vi "FRCts20_Backend_API_CompetitionRoot.vi"(8 "error in (no error)":errorcluster, 10 "Message":T1="GetCompetitionRoot") -> (0 "error out":errorcluster, 2 "Status":string, 3 "Competitions":T2)   [LabVIEW 2014]
doc: "This VI currently has just one command, which is to return all competitions. This cannot be rolled into another API VI, as no other VIs return competitions."
uses:
  FRCts20_Backend_API_CompetitionRoot.ctl
  FRCts20_Backend_API_Command_CompRoot.ctl
  FRCts20_Backend_FGVOperation.ctl
  FRCts20_Backend_Engine.lvlib
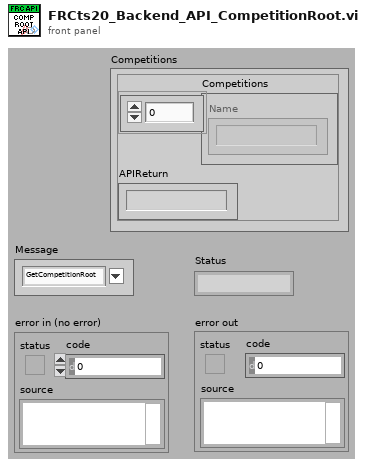
[diagram p1: front panel]
types:
  T1 = typedef "FRCts20_Backend_API_Command_CompRoot.ctl" = string
  T2 = typedef "FRCts20_Backend_API_CompetitionRoot.ctl" = cluster{"Competitions":string[], "APIReturn":string}
  T3 = typedef "FRCts20_Backend_Engine.lvlib/FRCts20_Backend_FGVOperation.ctl" = enum16{"Initialize", "EnqueueMessage", "EnqueueDataReturn", "FlushMessage", "FlushDataReturn"}
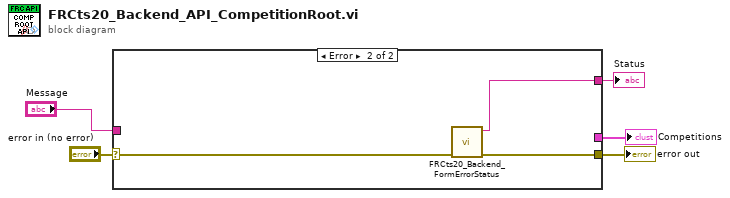
[diagram p0: block diagram]
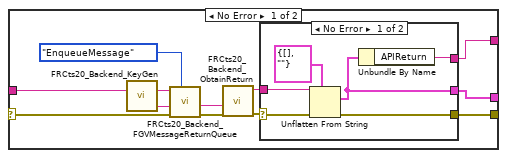
[diagram p2: hidden frame]
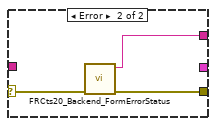
[diagram p3: hidden frame]
diagram:
  n1 = case shown="Error" "error in (no error)" {
    selector: "error in (no error)" -> [w16 w28]
    tunnel: [w7 w27] -> w4
    tunnel: [w9 w26] -> w3
    tunnel: [w8 _] -> w2
    tunnel: "Message" -> [w11 _]
    frame No Error {
      n2 = call "FRCts20_Backend_KeyGen.vi"() -> ("Keygen"=w15:string)  [unwired: 27 in]
      n3 = call "FRCts20_Backend_FGVMessageReturnQueue.vi"("Operation"=FRCts20_Backend_FGVOperation."EnqueueMessage", "error in (no error)"=w16, "Key"=w15, "Message Name"=w11) -> ("error out"=w13:errorcluster, "Key (Duplicate)"=w12:string)  [unwired: 6 in]
      n4 = call "FRCts20_Backend_ObtainReturn.vi"("error in (no error)"=w13, "Key"=w12) -> ("error out"=w10:errorcluster, "Message Value"=w6:string)  [unwired: 8 in]
      n5 = case shown="No Error" w10 {
        selector: w10 -> [w21 w23]
        tunnel: [w22 w24] -> w7
        tunnel: [w20 _] -> w8
        tunnel: [w19 w25] -> w9
        tunnel: w6 -> [w17 _]
        frame No Error {
          n6 = Unflatten From String(type=T2 {"Competitions"=[], "APIReturn"=""} ("Competitions"), binary string=w17, error in (no error)=w21) -> (value=w20:T2, error out=w22:errorcluster)  [unwired: 2 in, 1 out]
          n7 = Unbundle By Name(w20) -> ("APIReturn"=w19:string)
        }
        frame Error {
          n8 = call "FRCts20_Backend_FormErrorStatus.vi"("error in (no error)"=w23) -> ("error out"=w24:errorcluster, "String"=w25:string)  [unwired: 9 in]
        }
      }
    }
    frame Error {
      n9 = call "FRCts20_Backend_FormErrorStatus.vi"("error in (no error)"=w28) -> ("error out"=w27:errorcluster, "String"=w26:string)  [unwired: 9 in]
    }
  }
  "error out" <- w4
  "Status" <- w3
  "Competitions" <- w2
